vi "Диалог_на_Макро.vi"(8 "СОСТОЯНИЕ":bool, 11 "String":string) -> (3 "ВЫХОД":bool)   [LabVIEW 2016, in "Library.lvlib"]
uses:
  Granule-2000AT/PC/Library.lvlib
panel:
  in  "НЕТ":bool
  in  "ДА":bool
  out "ВОПРОС":string
  # "MAKRO"
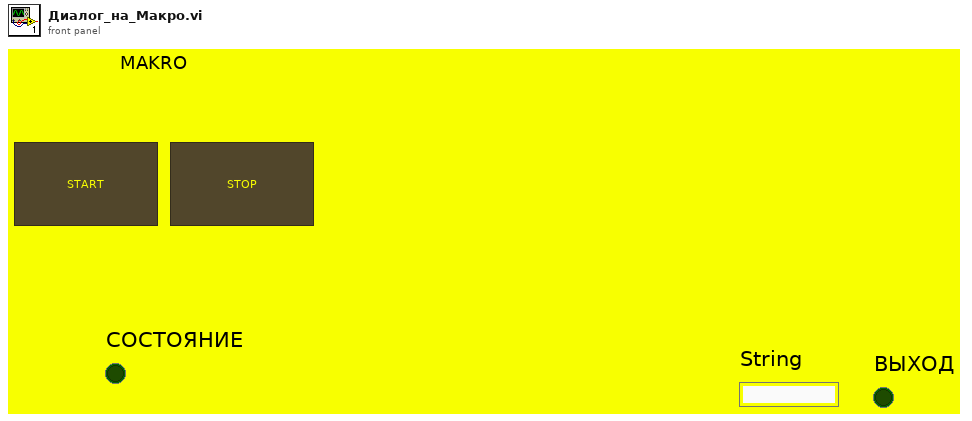
[diagram p1: front panel]
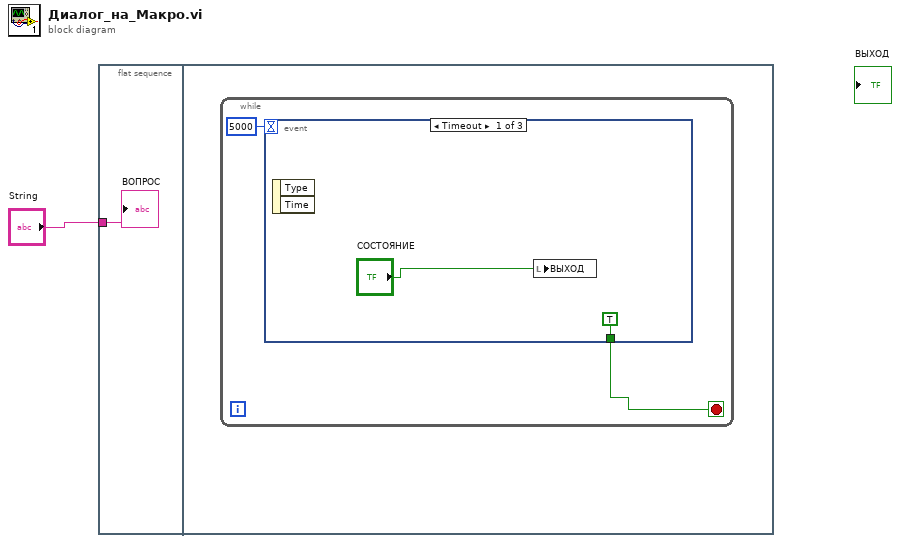
[diagram p0: block diagram]
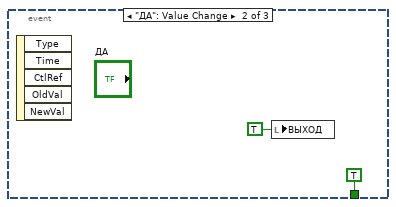
[diagram p2: hidden frame]
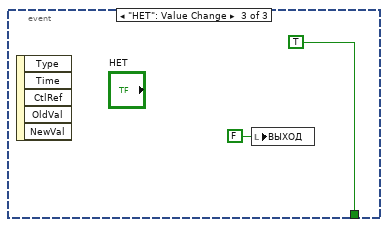
[diagram p3: hidden frame]
diagram:
  n1 = flat-sequence {
    tunnel: "String" -> [w2]
    frame #0 {
      "ВОПРОС" <- w2
    }
    frame #1 {
      n2 = while {
        stop <- w4 stop-if-true
        n3 = event shown="[0] Timeout" {
          selector: _ -> [_ _ _]
          dyn-events: _ -> [_ _ _]
          timeout: 5000 -> [_ _ _]
          tunnel: [TRUE ("Boolean") TRUE ("Boolean") TRUE ("Boolean")] -> w4
          event Timeout {
            n4 = event-data() -> ()  [unwired: 1 in, 2 out]
            n5 = local write "ВЫХОД"("СОСТОЯНИЕ") -> ()
          }
          event "ДА": Value Change {
            n6 = event-data() -> ()  [unwired: 1 in, 5 out]
            n7 = local write "ВЫХОД"(TRUE ("ВЫХОД")) -> ()
          }
          event "НЕТ": Value Change {
            n8 = event-data() -> ()  [unwired: 1 in, 5 out]
            n9 = local write "ВЫХОД"(FALSE ("ВЫХОД")) -> ()
          }
        }
      }
    }
  }
